vi "Front Panel Update Defer.vi"(6 "Close VI Reference? (T)":bool=TRUE, 8 "error in (no error)":errorcluster, 9 "Defer Panel Updates? (F)":bool, 10 "VI Reference (Calling VI)":refnum<vi>) -> (0 "error out":errorcluster)   [LabVIEW 2011]
doc: "This VI will defer or undefer front panel updates. Pass in the VI Reference to the VI to control. If none is passed in the calling VI will be used. To defer front panel updates, set <b>Defer Panel Updates</b> to TRUE. After doing this the VI will not have updates performed on the front panel until this VI is called again with <b>Defer Panel Updates</b> set to FALSE.\n\nOptionally set <b>Close VI Reference?</b>. By default it is TRUE and will close the VI reference passed in. If set to FALSE it will not close it.\n-------------\nBrian Hoover (hooovahh)"
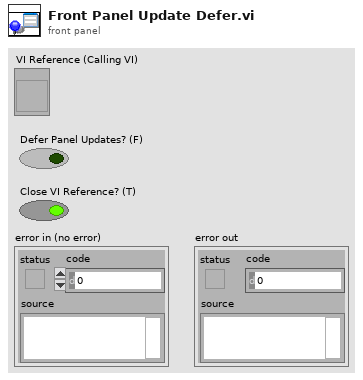
[diagram p1: front panel]
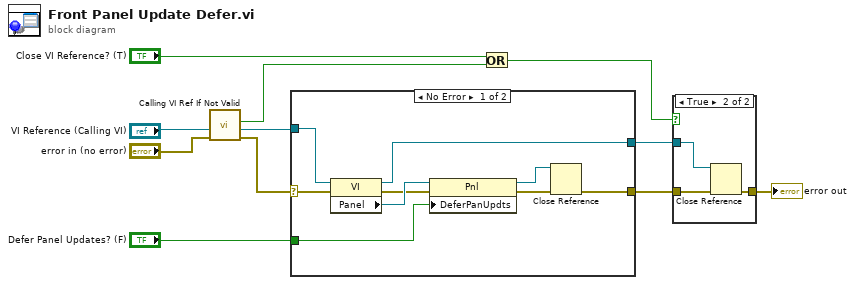
[diagram p0: block diagram]
diagram:
  n1 = call "Calling VI Ref If Not Valid.vi"("error in (no error)"="error in (no error)", "VI Reference"="VI Reference (Calling VI)") -> ("error out"=w7:errorcluster, "Valid VI Ref"=w9:refnum<vi>, "New Reference Opened"=w1:bool)  [unwired: 7 in]
  n2 = case shown="No Error" w7 {
    selector: w7 -> [w14 w22]
    tunnel: w9 -> [w16 w21]
    tunnel: "Defer Panel Updates? (F)" -> [w15 _]
    tunnel: [w13 w22] -> w6
    tunnel: [w12 w21] -> w3
    frame No Error {
      n3 = property class="VI"(reference=w16, error in=w14) -> (reference out=w12:refnum<vi>, error out=w19:errorcluster, "Panel"=w20:refnum<vi>)
      n4 = property class="Pnl"(reference=w20, error in=w19, "DeferPanUpdts"=w15) -> (reference out=w18:refnum<vi>, error out=w17:errorcluster)
      n5 = Close Reference(reference=w18, error in (no error)=w17) -> (error out=w13:errorcluster)
    }
    frame Error {
    }
  }
  n6 = Or(x="Close VI Reference? (T)", y=w1) -> (x .or. y?=w2:bool)
  n7 = case shown="True" w2 {
    tunnel: w3 -> [_ w26]
    tunnel: w6 -> [w23 w25]
    tunnel: [w23 w24] -> w5
    frame False {
    }
    frame True {
      n8 = Close Reference(reference=w26, error in (no error)=w25) -> (error out=w24:errorcluster)
    }
  }
  "error out" <- w5
